vi "FPGA Main.vi"() -> ()   [LabVIEW 2019]
uses:
  <vilib>/platform/TimedLoop/XDataNode/XDataNode.xnode
  <vilib>/Platform/TimedLoop/XDataNode/nitl_modes.ctl
  <vilib>/Platform/TimedLoop/XDataNode/XDNodeRunTimeDep.lvlib
  <vilib>/Platform/TimedLoop/XDataNode/wakeup.ctl
  <vilib>/Platform/TimedLoop/XDataNode/timing_clust.ctl
  Bank/Bank.lvclass
  LRUTS FPGA IP.lvlib
  Bank/Bank Type.ctl
  Connector Bank Types.ctl
  Bank/Discrete Acquisition Bank Indicator.ctl
  Bank/PWM Acquisition Channel Measurement.ctl
  Bank/PWM Acquisition Channel Results.ctl
  Bank/PWM Acquisition Bank Results.ctl
  Bank/PWM Acquisition Channel Settings.ctl
  Bank/PWM Acquisition Bank Settings.ctl
  Bank/Discrete Generation Bank Control.ctl
  Bank/PWM Generation Channel Settings.ctl
  Bank/PWM Generation Bank Settings.ctl
panel:
  out "Connector 0 Bank 3 Discrete Acquisition":T1
  out "Connector 0 Bank 2 Discrete Acquisition":T1
  out "Connector 0 Bank 1 Discrete Acquisition":T1
  out "Connector 0 Bank 0 Discrete Acquisition":T1
  in  "Connector 3 Bank 0 PWM Generation Settings":T2={"PWM 0 Settings"={"ACTIVE EDGE"=TRUE, "ACTIVE TICKS"=0, "INACTIVE TICKS"=0}, "PWM 1 Settings"={"ACTIVE EDGE"=TRUE, "ACTIVE TICKS"=0, "INACTIVE TICKS"=0}, "PWM 2 Settings"={"ACTIVE EDGE"=TRUE, "ACTIVE TICKS"=0, "INACTIVE TICKS"=0}, "PWM 3 Settings"={"ACTIVE EDGE"=TRUE, "ACTIVE TICKS"=0, "INACTIVE TICKS"=0}, "PWM 4 Settings"={"ACTIVE EDGE"=TRUE, "ACTIVE TICKS"=0, "INACTIVE TICKS"=0}, "PWM 5 Settings"={"ACTIVE EDGE"=TRUE, "ACTIVE TICKS"=0, "INACTIVE TICKS"=0}, "PWM 6 Settings"={"ACTIVE EDGE"=TRUE, "ACTIVE TICKS"=0, "INACTIVE TICKS"=0}, "PWM 7 Settings"={"ACTIVE EDGE"=TRUE, "ACTIVE TICKS"=0, "INACTIVE TICKS"=0}}
  in  "Connector 3 Bank 1 PWM Generation Settings":T2={"PWM 0 Settings"={"ACTIVE EDGE"=TRUE, "ACTIVE TICKS"=0, "INACTIVE TICKS"=0}, "PWM 1 Settings"={"ACTIVE EDGE"=TRUE, "ACTIVE TICKS"=0, "INACTIVE TICKS"=0}, "PWM 2 Settings"={"ACTIVE EDGE"=TRUE, "ACTIVE TICKS"=0, "INACTIVE TICKS"=0}, "PWM 3 Settings"={"ACTIVE EDGE"=TRUE, "ACTIVE TICKS"=0, "INACTIVE TICKS"=0}, "PWM 4 Settings"={"ACTIVE EDGE"=TRUE, "ACTIVE TICKS"=0, "INACTIVE TICKS"=0}, "PWM 5 Settings"={"ACTIVE EDGE"=TRUE, "ACTIVE TICKS"=0, "INACTIVE TICKS"=0}, "PWM 6 Settings"={"ACTIVE EDGE"=TRUE, "ACTIVE TICKS"=0, "INACTIVE TICKS"=0}, "PWM 7 Settings"={"ACTIVE EDGE"=TRUE, "ACTIVE TICKS"=0, "INACTIVE TICKS"=0}}
  in  "Connector 3 Bank 2 PWM Generation Settings":T2={"PWM 0 Settings"={"ACTIVE EDGE"=TRUE, "ACTIVE TICKS"=0, "INACTIVE TICKS"=0}, "PWM 1 Settings"={"ACTIVE EDGE"=TRUE, "ACTIVE TICKS"=0, "INACTIVE TICKS"=0}, "PWM 2 Settings"={"ACTIVE EDGE"=TRUE, "ACTIVE TICKS"=0, "INACTIVE TICKS"=0}, "PWM 3 Settings"={"ACTIVE EDGE"=TRUE, "ACTIVE TICKS"=0, "INACTIVE TICKS"=0}, "PWM 4 Settings"={"ACTIVE EDGE"=TRUE, "ACTIVE TICKS"=0, "INACTIVE TICKS"=0}, "PWM 5 Settings"={"ACTIVE EDGE"=TRUE, "ACTIVE TICKS"=0, "INACTIVE TICKS"=0}, "PWM 6 Settings"={"ACTIVE EDGE"=TRUE, "ACTIVE TICKS"=0, "INACTIVE TICKS"=0}, "PWM 7 Settings"={"ACTIVE EDGE"=TRUE, "ACTIVE TICKS"=0, "INACTIVE TICKS"=0}}
  in  "Connector 3 Bank 3 PWM Generation Settings":T2={"PWM 0 Settings"={"ACTIVE EDGE"=TRUE, "ACTIVE TICKS"=0, "INACTIVE TICKS"=0}, "PWM 1 Settings"={"ACTIVE EDGE"=TRUE, "ACTIVE TICKS"=0, "INACTIVE TICKS"=0}, "PWM 2 Settings"={"ACTIVE EDGE"=TRUE, "ACTIVE TICKS"=0, "INACTIVE TICKS"=0}, "PWM 3 Settings"={"ACTIVE EDGE"=TRUE, "ACTIVE TICKS"=0, "INACTIVE TICKS"=0}, "PWM 4 Settings"={"ACTIVE EDGE"=TRUE, "ACTIVE TICKS"=0, "INACTIVE TICKS"=0}, "PWM 5 Settings"={"ACTIVE EDGE"=TRUE, "ACTIVE TICKS"=0, "INACTIVE TICKS"=0}, "PWM 6 Settings"={"ACTIVE EDGE"=TRUE, "ACTIVE TICKS"=0, "INACTIVE TICKS"=0}, "PWM 7 Settings"={"ACTIVE EDGE"=TRUE, "ACTIVE TICKS"=0, "INACTIVE TICKS"=0}}
  in  "Connector 2 Bank 3 Discrete Stimulus":T4
  in  "Connector 2 Bank 2 Discrete Stimulus":T4
  in  "Connector 2 Bank 1 Discrete Stimulus":T4
  in  "Connector 2 Bank 0 Discrete Stimulus":T4
  in  "Connector 1 Bank 3 Settings":T5={"PWM 0 Settings"={"ACTIVE EDGE"=TRUE, "TIMEOUT"=40000000}, "PWM 1 Settings"={"ACTIVE EDGE"=TRUE, "TIMEOUT"=40000000}, "PWM 2 Settings"={"ACTIVE EDGE"=TRUE, "TIMEOUT"=40000000}, "PWM 3 Settings"={"ACTIVE EDGE"=TRUE, "TIMEOUT"=40000000}, "PWM 4 Settings"={"ACTIVE EDGE"=TRUE, "TIMEOUT"=40000000}, "PWM 5 Settings"={"ACTIVE EDGE"=TRUE, "TIMEOUT"=40000000}, "PWM 6 Settings"={"ACTIVE EDGE"=TRUE, "TIMEOUT"=40000000}, "PWM 7 Settings"={"ACTIVE EDGE"=TRUE, "TIMEOUT"=40000000}}
  in  "Connector 1 Bank 2 Settings":T5={"PWM 0 Settings"={"ACTIVE EDGE"=TRUE, "TIMEOUT"=40000000}, "PWM 1 Settings"={"ACTIVE EDGE"=TRUE, "TIMEOUT"=40000000}, "PWM 2 Settings"={"ACTIVE EDGE"=TRUE, "TIMEOUT"=40000000}, "PWM 3 Settings"={"ACTIVE EDGE"=TRUE, "TIMEOUT"=40000000}, "PWM 4 Settings"={"ACTIVE EDGE"=TRUE, "TIMEOUT"=40000000}, "PWM 5 Settings"={"ACTIVE EDGE"=TRUE, "TIMEOUT"=40000000}, "PWM 6 Settings"={"ACTIVE EDGE"=TRUE, "TIMEOUT"=40000000}, "PWM 7 Settings"={"ACTIVE EDGE"=TRUE, "TIMEOUT"=40000000}}
  in  "Connector 1 Bank 1 Settings":T5={"PWM 0 Settings"={"ACTIVE EDGE"=TRUE, "TIMEOUT"=40000000}, "PWM 1 Settings"={"ACTIVE EDGE"=TRUE, "TIMEOUT"=40000000}, "PWM 2 Settings"={"ACTIVE EDGE"=TRUE, "TIMEOUT"=40000000}, "PWM 3 Settings"={"ACTIVE EDGE"=TRUE, "TIMEOUT"=40000000}, "PWM 4 Settings"={"ACTIVE EDGE"=TRUE, "TIMEOUT"=40000000}, "PWM 5 Settings"={"ACTIVE EDGE"=TRUE, "TIMEOUT"=40000000}, "PWM 6 Settings"={"ACTIVE EDGE"=TRUE, "TIMEOUT"=40000000}, "PWM 7 Settings"={"ACTIVE EDGE"=TRUE, "TIMEOUT"=40000000}}
  in  "Connector 1 Bank 0 Settings":T5={"PWM 0 Settings"={"ACTIVE EDGE"=TRUE, "TIMEOUT"=40000000}, "PWM 1 Settings"={"ACTIVE EDGE"=TRUE, "TIMEOUT"=40000000}, "PWM 2 Settings"={"ACTIVE EDGE"=TRUE, "TIMEOUT"=40000000}, "PWM 3 Settings"={"ACTIVE EDGE"=TRUE, "TIMEOUT"=40000000}, "PWM 4 Settings"={"ACTIVE EDGE"=TRUE, "TIMEOUT"=40000000}, "PWM 5 Settings"={"ACTIVE EDGE"=TRUE, "TIMEOUT"=40000000}, "PWM 6 Settings"={"ACTIVE EDGE"=TRUE, "TIMEOUT"=40000000}, "PWM 7 Settings"={"ACTIVE EDGE"=TRUE, "TIMEOUT"=40000000}}
  out "Connector 1 Bank 3 PWM Acquisition":T7
  out "Connector 1 Bank 2 PWM Acquisition":T7
  out "Connector 1 Bank 1 PWM Acquisition":T7
  out "Connector 1 Bank 0 PWM Acquisition":T7
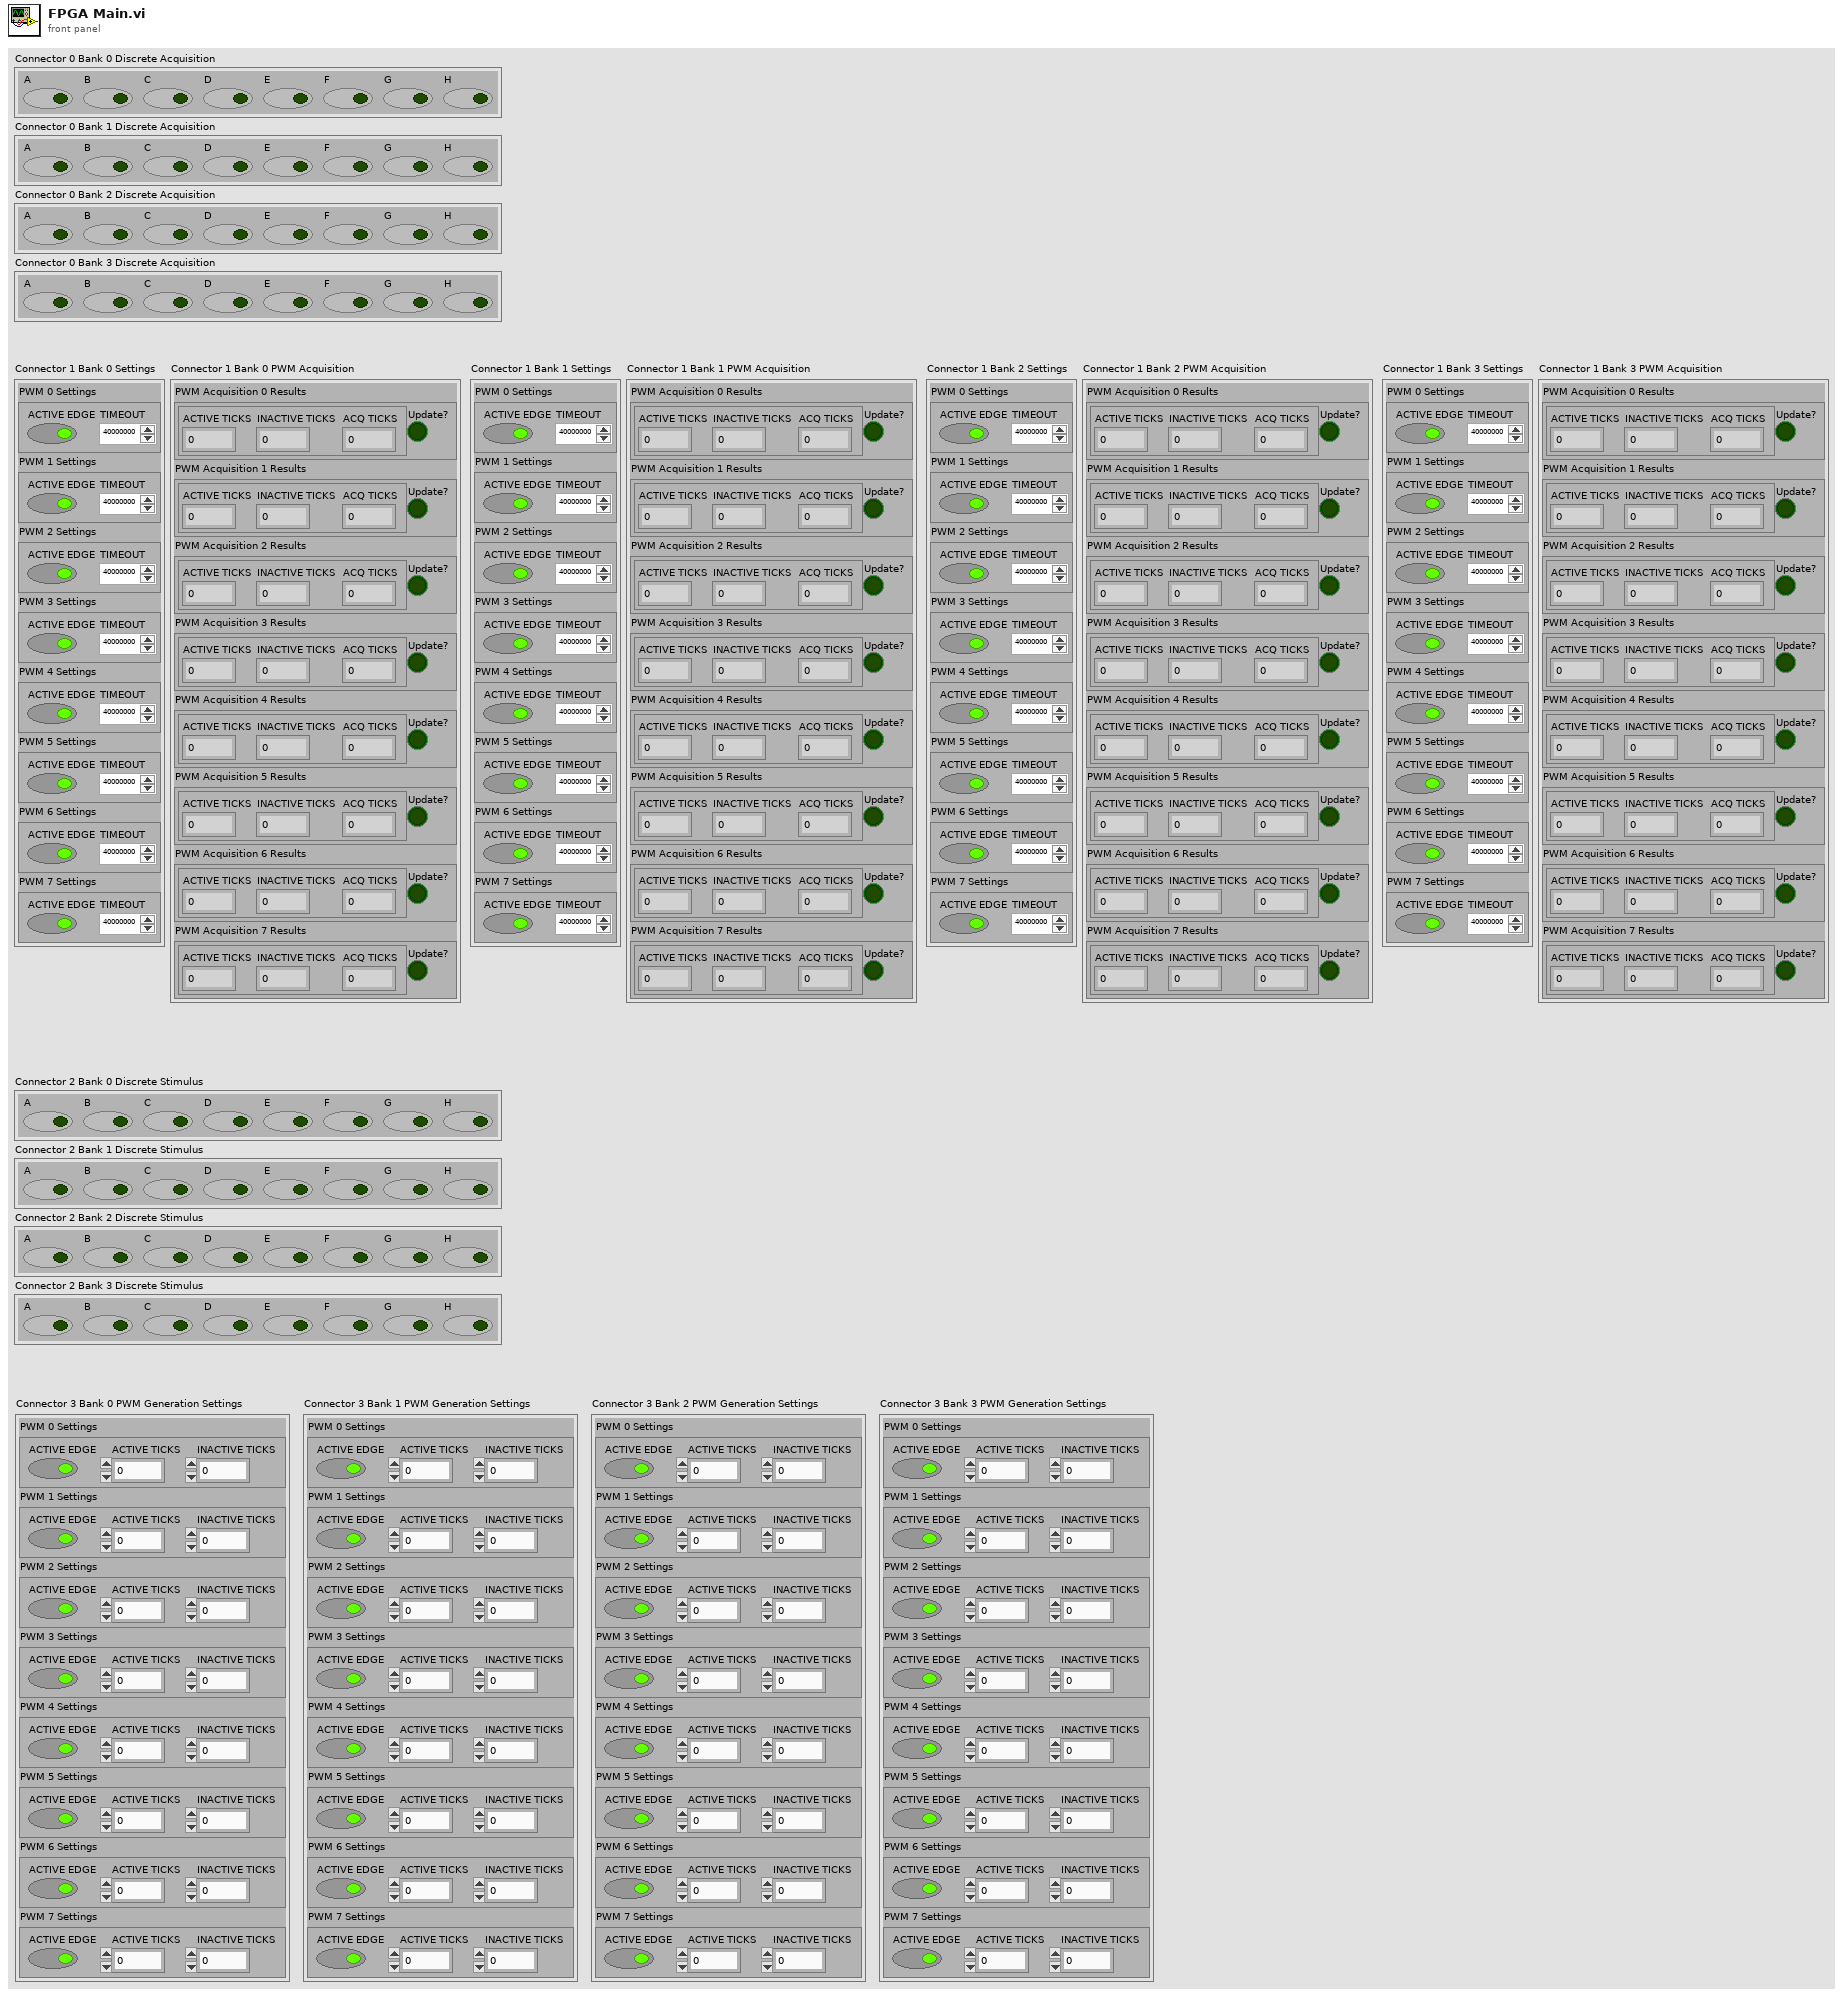
[diagram p1: front panel]
types:
  T1 = typedef "LRUTS FPGA IP.lvlib/Bank.lvclass/Discrete Acquisition Bank Indicator.ctl" = cluster{"A":bool, "B":bool, "C":bool, "D":bool, "E":bool, "F":bool, "G":bool, "H":bool}
  T2 = typedef "LRUTS FPGA IP.lvlib/Bank.lvclass/PWM Generation Bank Settings.ctl" = cluster{"PWM 0 Settings":T3, "PWM 1 Settings":T3, "PWM 2 Settings":T3, "PWM 3 Settings":T3, "PWM 4 Settings":T3, "PWM 5 Settings":T3, "PWM 6 Settings":T3, "PWM 7 Settings":T3}
  T3 = typedef "LRUTS FPGA IP.lvlib/Bank.lvclass/PWM Generation Channel Settings.ctl" = cluster{"ACTIVE EDGE":bool, "ACTIVE TICKS":u32, "INACTIVE TICKS":u32}
  T4 = typedef "LRUTS FPGA IP.lvlib/Bank.lvclass/Discrete Generation Bank Control.ctl" = cluster{"A":bool, "B":bool, "C":bool, "D":bool, "E":bool, "F":bool, "G":bool, "H":bool}
  T5 = typedef "LRUTS FPGA IP.lvlib/Bank.lvclass/PWM Acquisition Bank Settings.ctl" = cluster{"PWM 0 Settings":T6, "PWM 1 Settings":T6, "PWM 2 Settings":T6, "PWM 3 Settings":T6, "PWM 4 Settings":T6, "PWM 5 Settings":T6, "PWM 6 Settings":T6, "PWM 7 Settings":T6}
  T6 = typedef "LRUTS FPGA IP.lvlib/Bank.lvclass/PWM Acquisition Channel Settings.ctl" = cluster{"ACTIVE EDGE":bool, "TIMEOUT":u32}
  T7 = typedef "LRUTS FPGA IP.lvlib/Bank.lvclass/PWM Acquisition Bank Results.ctl" = cluster{"PWM Acquisition 0 Results":T8, "PWM Acquisition 1 Results":T8, "PWM Acquisition 2 Results":T8, "PWM Acquisition 3 Results":T8, "PWM Acquisition 4 Results":T8, "PWM Acquisition 5 Results":T8, "PWM Acquisition 6 Results":T8, "PWM Acquisition 7 Results":T8}
  T8 = typedef "LRUTS FPGA IP.lvlib/Bank.lvclass/PWM Acquisition Channel Results.ctl" = cluster{"Measurement":T9, "Update?":bool}
  T9 = typedef "LRUTS FPGA IP.lvlib/Bank.lvclass/PWM Acquisition Channel Measurement.ctl" = cluster{"ACTIVE TICKS":u32, "INACTIVE TICKS":u32, "ACQ TICKS":u32}
  T10 = typedef "LRUTS FPGA IP.lvlib/Connector Bank Types.ctl" = cluster{"Bank 0 type":T11, "Bank 1 type":T11, "Bank 2 type":T11, "Bank 3 type":T11}
  T11 = typedef "LRUTS FPGA IP.lvlib/Bank.lvclass/Bank Type.ctl" = enum16{"None", "Discrete Acquisition", "Discrete Generation", "PWM Acquisition", "PWM Generation"}
  T12 = typedef "XDNodeRunTimeDep.lvlib/timing_clust.ctl" = cluster{"Expected End [f-1]":u64, "Actual End [f-1]":u64, "Finished Late? [f-1]":bool, "Expected End [i-1]":u64, "Actual End [i-1]":u64, "Finished Late? [i-1]":bool, "Expected Start [i]":u64, "Actual Start [i]":u64, "Expected Start [f]":u64, "Actual Start [f]":u64, "Source Name":string, "Structure Name":string, "Period":i64, "Deadline":i64, "Offset":i64, "Start":i64, "Priority":i32, "Timeout":i32, "Mode":T13, "Wakeup Reason":T14, "Error":errorcluster, "Source Type":string, "Secondary Source Type":string, "Global End Time":u64, "Global Start Time":u64, "Frame Duration":u64, "Iteration Duration":u64, "Assigned CPU":i32, "I/O Scan Engine Mode":u32}
  T13 = typedef "XDNodeRunTimeDep.lvlib/nitl_modes.ctl" = enum32{"No Change", "Process missed periods, maintain original phase", "Discard missed periods, maintain original phase", "Process missed periods, ignore original phase", "Discard missed periods, ignore original phase"}
  T14 = typedef "XDNodeRunTimeDep.lvlib/wakeup.ctl" = enum32{"Normal", "Aborted", "Asynchronous wakeup", "Timing source error", "Timed loop error", "Timeout"}
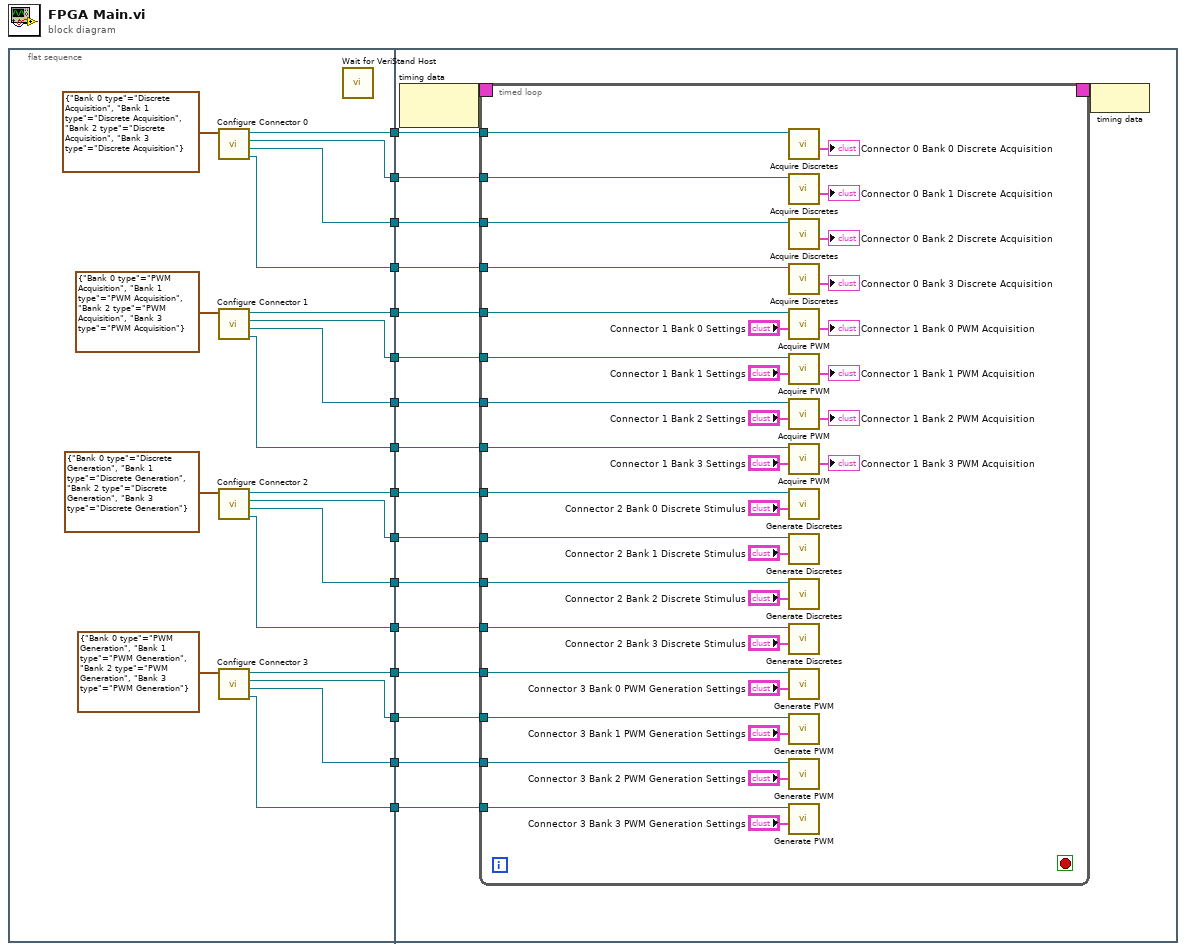
[diagram p0: block diagram]
diagram:
  n1 = flat-sequence {
    tunnel: [w35] -> w16
    tunnel: [w34] -> w15
    tunnel: [w33] -> w14
    tunnel: [w32] -> w13
    tunnel: [w28] -> w12
    tunnel: [w27] -> w11
    tunnel: [w26] -> w10
    tunnel: [w25] -> w9
    tunnel: [w24] -> w8
    tunnel: [w23] -> w7
    tunnel: [w22] -> w6
    tunnel: [w21] -> w5
    tunnel: [w20] -> w4
    tunnel: [w19] -> w3
    tunnel: [w18] -> w2
    tunnel: [w17] -> w1
    tunnel: w16 -> [w52]
    tunnel: w15 -> [w51]
    tunnel: w14 -> [w50]
    tunnel: w13 -> [w49]
    tunnel: w12 -> [w48]
    tunnel: w11 -> [w47]
    tunnel: w10 -> [w46]
    tunnel: w9 -> [w45]
    tunnel: w8 -> [w44]
    tunnel: w7 -> [w43]
    tunnel: w6 -> [w42]
    tunnel: w5 -> [w41]
    tunnel: w4 -> [w40]
    tunnel: w3 -> [w39]
    tunnel: w2 -> [w38]
    tunnel: w1 -> [w37]
    frame #0 {
      n2 = call "Configure Connector 0.vi"("Bank Types"=T10 {"Bank 0 type"=enum."Discrete Acquisition", "Bank 1 type"=enum."Discrete Acquisition", "Bank 2 type"=enum."Discrete Acquisition", "Bank 3 type"=enum."Discrete Acquisition"}) -> ("Connector 0 Bank 3 out"=w32:refnum<class "Bank.lvclass">, "Connector 0 Bank 2 out"=w33:refnum<class "Bank.lvclass">, "Connector 0 Bank 1 out"=w34:refnum<class "Bank.lvclass">, "Connector 0 Bank 0 out"=w35:refnum<class "Bank.lvclass">)  [unwired: 7 in]
      n3 = call "Configure Connector 1.vi"("Bank Types"=T10 {"Bank 0 type"=enum."PWM Acquisition", "Bank 1 type"=enum."PWM Acquisition", "Bank 2 type"=enum."PWM Acquisition", "Bank 3 type"=enum."PWM Acquisition"}) -> ("Connector 0 Bank 3 out"=w25:refnum<class "Bank.lvclass">, "Connector 0 Bank 2 out"=w26:refnum<class "Bank.lvclass">, "Connector 0 Bank 1 out"=w27:refnum<class "Bank.lvclass">, "Connector 0 Bank 0 out"=w28:refnum<class "Bank.lvclass">)  [unwired: 7 in]
      n4 = call "Configure Connector 2.vi"("Bank Types"=T10 {"Bank 0 type"=enum."Discrete Generation", "Bank 1 type"=enum."Discrete Generation", "Bank 2 type"=enum."Discrete Generation", "Bank 3 type"=enum."Discrete Generation"}) -> ("Connector 0 Bank 3 out"=w21:refnum<class "Bank.lvclass">, "Connector 0 Bank 2 out"=w22:refnum<class "Bank.lvclass">, "Connector 0 Bank 1 out"=w23:refnum<class "Bank.lvclass">, "Connector 0 Bank 0 out"=w24:refnum<class "Bank.lvclass">)  [unwired: 7 in]
      n5 = call "Configure Connector 3.vi"("Bank Types"=T10 {"Bank 0 type"=enum."PWM Generation", "Bank 1 type"=enum."PWM Generation", "Bank 2 type"=enum."PWM Generation", "Bank 3 type"=enum."PWM Generation"}) -> ("Connector 0 Bank 3 out"=w17:refnum<class "Bank.lvclass">, "Connector 0 Bank 2 out"=w18:refnum<class "Bank.lvclass">, "Connector 0 Bank 1 out"=w19:refnum<class "Bank.lvclass">, "Connector 0 Bank 0 out"=w20:refnum<class "Bank.lvclass">)  [unwired: 7 in]
      n6 = call "Wait for VeriStand Host.vi"() -> ()  [unwired: 12 in]
    }
    frame #1 {
      n7 = node-c288() -> (w54:T12)  [unwired: 1 in]
      n8 = timed-loop {
        timing: w54 -> [_]
        timing-out: [_] -> w53
        tunnel: w52 -> [w90]
        tunnel: w51 -> [w89]
        tunnel: w50 -> [w88]
        tunnel: w49 -> [w87]
        tunnel: w48 -> [w86]
        tunnel: w47 -> [w85]
        tunnel: w46 -> [w84]
        tunnel: w45 -> [w83]
        tunnel: w44 -> [w82]
        tunnel: w43 -> [w81]
        tunnel: w42 -> [w80]
        tunnel: w41 -> [w79]
        tunnel: w40 -> [w78]
        tunnel: w39 -> [w77]
        tunnel: w38 -> [w76]
        tunnel: w37 -> [w75]
        stop <- _ stop-if-true
        n9 = call "Acquire Discretes.vi"("Bank in"=w90) -> ("Connector m Bank n Discrete Acquisition"=→"Connector 0 Bank 0 Discrete Acquisition":T1)  [unwired: 9 in, 1 out]
        n10 = call "Acquire Discretes.vi"("Bank in"=w89) -> ("Connector m Bank n Discrete Acquisition"=→"Connector 0 Bank 1 Discrete Acquisition":T1)  [unwired: 9 in, 1 out]
        n11 = call "Acquire Discretes.vi"("Bank in"=w88) -> ("Connector m Bank n Discrete Acquisition"=→"Connector 0 Bank 2 Discrete Acquisition":T1)  [unwired: 9 in, 1 out]
        n12 = call "Acquire Discretes.vi"("Bank in"=w87) -> ("Connector m Bank n Discrete Acquisition"=→"Connector 0 Bank 3 Discrete Acquisition":T1)  [unwired: 9 in, 1 out]
        n13 = call "Acquire PWM.vi"("Connector m Bank n Settings"="Connector 1 Bank 0 Settings", "Bank in"=w86) -> ("Connector m Bank n PWM Acquisition"=→"Connector 1 Bank 0 PWM Acquisition":T7)  [unwired: 8 in, 1 out]
        n14 = call "Acquire PWM.vi"("Connector m Bank n Settings"="Connector 1 Bank 1 Settings", "Bank in"=w85) -> ("Connector m Bank n PWM Acquisition"=→"Connector 1 Bank 1 PWM Acquisition":T7)  [unwired: 8 in, 1 out]
        n15 = call "Acquire PWM.vi"("Connector m Bank n Settings"="Connector 1 Bank 2 Settings", "Bank in"=w84) -> ("Connector m Bank n PWM Acquisition"=→"Connector 1 Bank 2 PWM Acquisition":T7)  [unwired: 8 in, 1 out]
        n16 = call "Acquire PWM.vi"("Connector m Bank n Settings"="Connector 1 Bank 3 Settings", "Bank in"=w83) -> ("Connector m Bank n PWM Acquisition"=→"Connector 1 Bank 3 PWM Acquisition":T7)  [unwired: 8 in, 1 out]
        n17 = call "Generate Discretes.vi"("Connector m Bank n Discrete Stimulus"="Connector 2 Bank 0 Discrete Stimulus", "Bank in"=w82) -> ()  [unwired: 9 in, 1 out]
        n18 = call "Generate Discretes.vi"("Connector m Bank n Discrete Stimulus"="Connector 2 Bank 1 Discrete Stimulus", "Bank in"=w81) -> ()  [unwired: 9 in, 1 out]
        n19 = call "Generate Discretes.vi"("Connector m Bank n Discrete Stimulus"="Connector 2 Bank 2 Discrete Stimulus", "Bank in"=w80) -> ()  [unwired: 9 in, 1 out]
        n20 = call "Generate Discretes.vi"("Connector m Bank n Discrete Stimulus"="Connector 2 Bank 3 Discrete Stimulus", "Bank in"=w79) -> ()  [unwired: 9 in, 1 out]
        n21 = call "Generate PWM.vi"("Connector m Bank n PWM Generation Settings"="Connector 3 Bank 0 PWM Generation Settings", "Bank in"=w78) -> ()  [unwired: 9 in, 1 out]
        n22 = call "Generate PWM.vi"("Connector m Bank n PWM Generation Settings"="Connector 3 Bank 1 PWM Generation Settings", "Bank in"=w77) -> ()  [unwired: 9 in, 1 out]
        n23 = call "Generate PWM.vi"("Connector m Bank n PWM Generation Settings"="Connector 3 Bank 2 PWM Generation Settings", "Bank in"=w76) -> ()  [unwired: 9 in, 1 out]
        n24 = call "Generate PWM.vi"("Connector m Bank n PWM Generation Settings"="Connector 3 Bank 3 PWM Generation Settings", "Bank in"=w75) -> ()  [unwired: 9 in, 1 out]
      }
      n25 = node-c288(w53) -> ()
    }
  }
